vi "BRig_dataLC_Cue_PostR_nRew1_l1.vi"() -> (2 "output_Cue_PostR_nRew1_l1":i32)   [LabVIEW 2014]
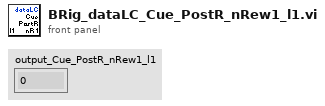
[diagram p1: front panel]
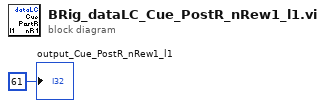
[diagram p0: block diagram]
diagram:
  "output_Cue_PostR_nRew1_l1" <- 61 ("output_iBlock")
